vi "14- Remove trailing space.vi"() -> ()   [LabVIEW 2019]
panel:
  out "Output string":string
  in  "Input string":string
  # "REMOVE TRAILING SPACE FROM INPUT STRING"
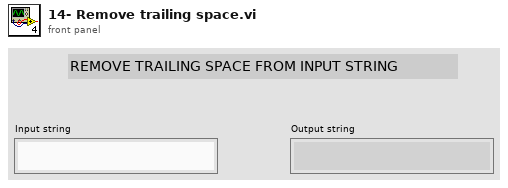
[diagram p1: front panel]
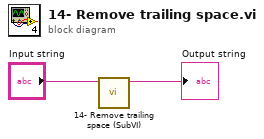
[diagram p0: block diagram]
diagram:
  n1 = call "14- Remove trailing space (SubVI).vi"("iNPUT STRING"="Input string") -> ("oUTPUT STRING"=→"Output string":string)  [unwired: 10 in]
